vi "Move and wait.vi"(5 "Device model":string, 7 "Resolution":dbl, 8 "error in (no error)":errorcluster, 9 "Position":cluster{"M1 pos":dbl, "M2 pos ":dbl}, 10 "Direction":T2, 11 "Module ID":i32) -> (0 "error out":errorcluster, 1 "Steps taken":i32, 2 "Position out":cluster{"M1 pos":dbl, "M2 pos ":dbl})   [LabVIEW 2020]
uses:
  NI_DAQ/Libraries/NI DAQ/NI DAQ.lvlib
  NI_DAQ/Libraries/NI DAQ/Support/Task list.ctl
  Controls/Motor controls---typedef.ctl
  controls/Motor direction ---typedef.ctl
panel:
  out "data":dbl[](array[numeric])
  in  "Motor control":T1={"EN1"=FALSE, "DIR1"=TRUE, "EN2"=FALSE, "DIR2"=TRUE, "TOG"=FALSE}
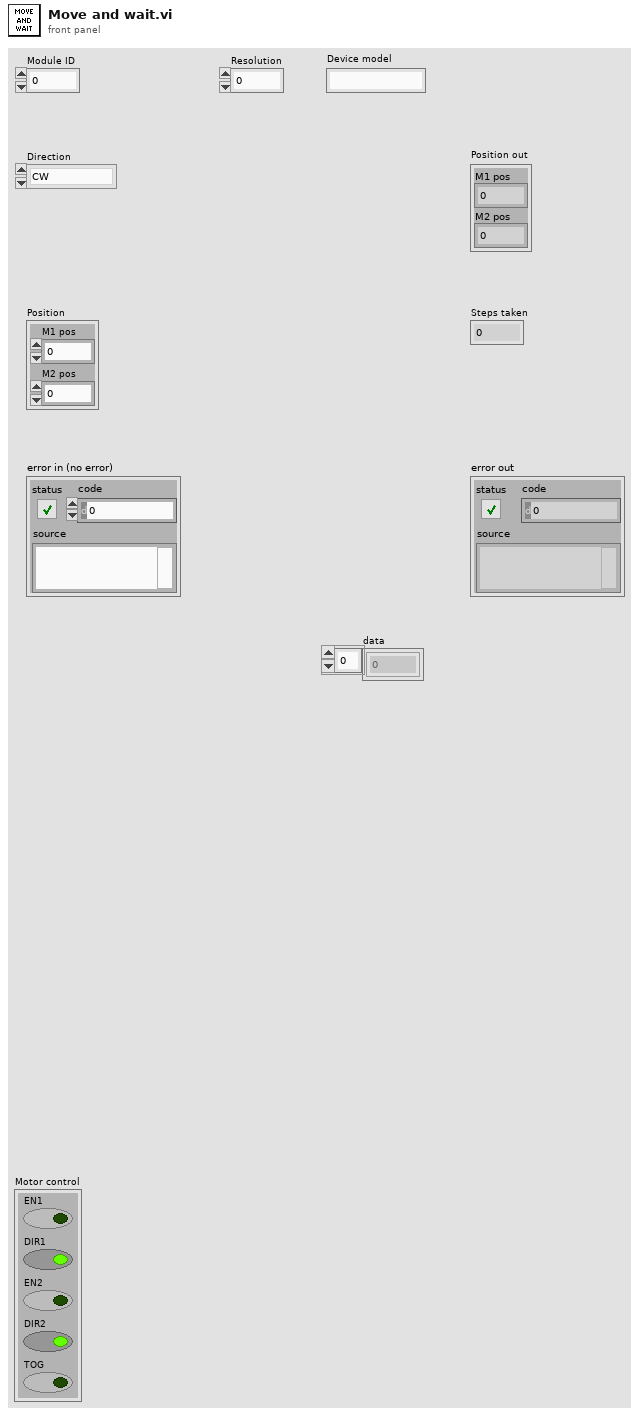
[diagram p1: front panel]
types:
  T1 = typedef "Motor controls---typedef.ctl" = cluster{"EN1":bool, "DIR1":bool, "EN2":bool, "DIR2":bool, "TOG":bool}
  T2 = typedef "Motor direction ---typedef.ctl" = enum16{"CW", "CCW", "IDLE"}
  T3 = typedef "NI DAQ.lvlib/Task list.ctl" = enum16{"All", "DO task", "DI task", "AO task", "AI task", "CI task", "CO task", "TC task"}
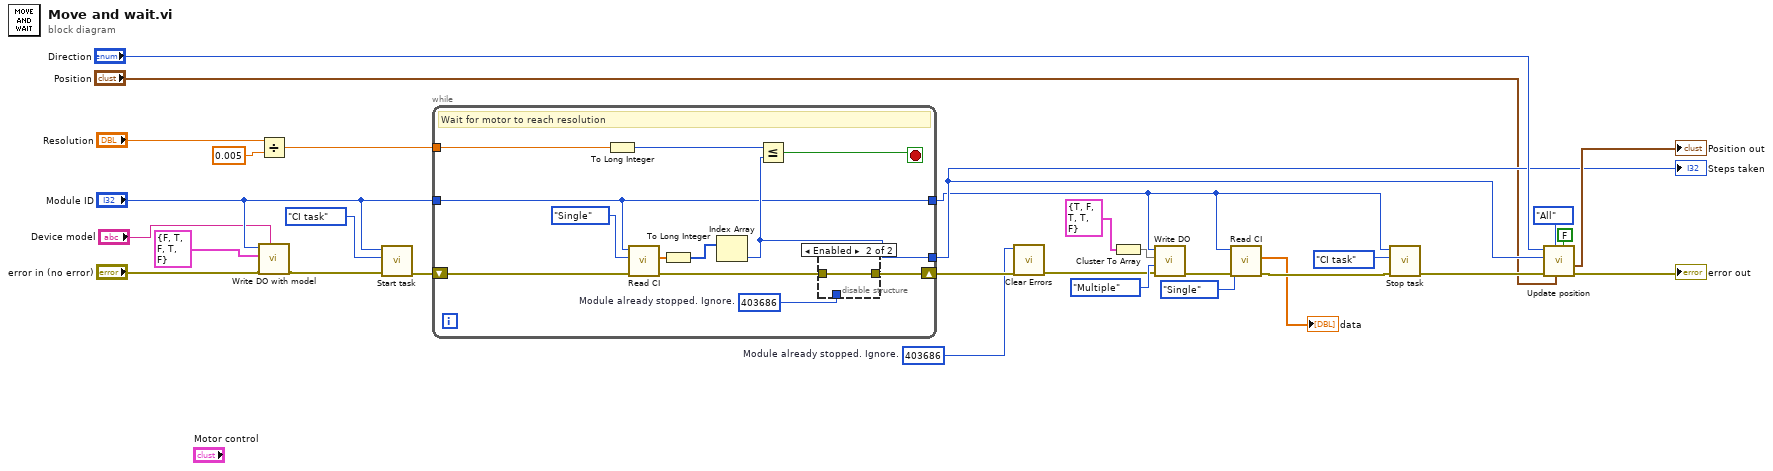
[diagram p0: block diagram]
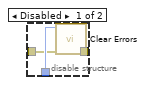
[diagram p2: hidden frame]
diagram:
  w2 = 403686  # Module already stopped. Ignore.
  n1 = Divide(x="Resolution", y=0.005) -> (x/y=w26:dbl)
  n2 = call "Write DO with model.vi"("Device model"="Device model", "error in"="error in (no error)", "Motor control"=T1 {"EN1"=FALSE, "DIR1"=TRUE, "EN2"=FALSE, "DIR2"=TRUE, "TOG"=FALSE}, "Module ID"="Module ID") -> ("error out"=w16:errorcluster)  [unwired: 7 in]
  n3 = call "Start task.vi"("error in"=w16, "Task list"=Task_list."CI task", "Module ID"="Module ID") -> ("error out"=w28:errorcluster)  [unwired: 8 in]
  n4 = while {
    tunnel: "Module ID" -> [w35]
    shift-right: [w34] -> w4
    shift-left: w28 -> [w42]
    tunnel: w26 -> [w38]
    tunnel: [w36] -> w12
    tunnel: [w35] -> w7
    stop <- w32 stop-if-true
    w33 = 403686  # Module already stopped. Ignore.
    # "Wait for motor to reach resolution"
    n5 = To Long Integer(number=w38) -> (32bit integer=w37:i32)
    n6 = call "Read CI.vi"("error in"=w42, "Samples"=enum16{"Single", "Multiple"}."Single", "Module ID"=w35) -> ("error out"=w31:errorcluster, "data"=w40:dbl[])  [unwired: 6 in, 1 out]
    n7 = To Long Integer(number=w40) -> (32bit integer=w39:i32[])
    n8 = Index Array(array=w39) -> (element=w36:i32)  [unwired: 1 in]
    n9 = Less Or Equal?(x=w37, y=w36) -> (x <= y?=w32:bool)
    n10 = disable-structure shown="Enabled" {
      disable-tunnel: [w45 w46] -> w34
      disable-tunnel: w33 -> [w44 _]
      disable-tunnel: w31 -> [w43 w46]
      frame Disabled {
        n11 = call <vilib>:"Clear Errors.vi"("error in (no error)"=w43, "specific error code to clear (0: all)"=w44) -> ("error out"=w45:errorcluster)  [unwired: 4 in, 1 out]
      }
      frame Enabled {
      }
    }
  }
  "Steps taken" <- w12
  n12 = call <vilib>:"Clear Errors.vi"("error in (no error)"=w4, "specific error code to clear (0: all)"=w2) -> ("error out"=w3:errorcluster)  [unwired: 4 in, 1 out]
  n13 = Cluster To Array(cluster=T1 {"EN1"=TRUE, "DIR1"=FALSE, "EN2"=TRUE, "DIR2"=TRUE, "TOG"=FALSE} ("Motor control")) -> (array=w20:bool[])
  n14 = call "Write DO.vi"("error in"=w3, "Samples"=enum16{"Single", "Multiple"}."Multiple", "Data"=w20, "Module ID"=w7) -> ("error out"=w9:errorcluster)  [unwired: 7 in]
  n15 = call "Read CI.vi"("error in"=w9, "Samples"=enum16{"Single", "Multiple"}."Single", "Module ID"=w7) -> ("error out"=w8:errorcluster, "data"=→"data":dbl[])  [unwired: 6 in, 1 out]
  n16 = call "Stop task.vi"("error in"=w8, "Task list"=Task_list."CI task", "Module ID"=w7) -> ("error out"=w10:errorcluster)  [unwired: 8 in]
  n17 = call "Update position.vi"("Acquiring?"=FALSE ("Homing?"), "Position 0"="Position", "Motor"=enum16{"All", "M1", "M2"}."All", "error in (no error)"=w10, "Direction M2"=w12, "Direction M1"="Direction") -> ("error out"=→"error out":errorcluster, "Position out"=→"Position out":cluster{"M1 pos":dbl, "M2 pos ":dbl})  [unwired: 4 in]
